vi "Initialize HMM Model.vi"(10 "M #observed states":i32=2, 11 "N #hidden states":i32=2) -> (3 "Init HMM":T1)   [LabVIEW 2014, in "HMM.lvlib"]
doc: "Generates the inital HMM a, b and Pi. The probability is random."
uses:
  HMM.lvlib
  Control/HMM Cluster.ctl
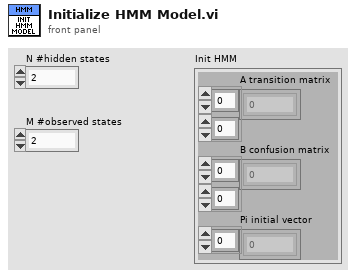
[diagram p1: front panel]
types:
  T1 = typedef "HMM.lvlib/HMM Cluster.ctl" = cluster{"A transition matrix":dbl[][], "B confusion matrix":dbl[][], "Pi initial vector":dbl[]}
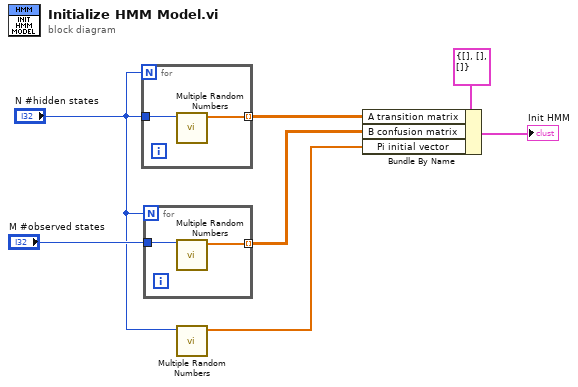
[diagram p0: block diagram]
diagram:
  n1 = for {
    N: "N #hidden states" -> [_]
    tunnel: "N #hidden states" -> [w9]
    tunnel: [w8] -> w5 mode=indexing
    n2 = call "Multiple Random Numbers.vi"("No. of rands"=w9) -> ("Random numbers"=w8:dbl[])  [unwired: 10 in]
  }
  n3 = for {
    N: "N #hidden states" -> [_]
    tunnel: "M #observed states" -> [w11]
    tunnel: [w10] -> w3 mode=indexing
    n4 = call "Multiple Random Numbers.vi"("No. of rands"=w11) -> ("Random numbers"=w10:dbl[])  [unwired: 10 in]
  }
  n5 = call "Multiple Random Numbers.vi"("No. of rands"="N #hidden states") -> ("Random numbers"=w1:dbl[])  [unwired: 10 in]
  n6 = Bundle By Name(cluster=T1 {"A transition matrix"=[], "B confusion matrix"=[], "Pi initial vector"=[]} ("Init lambda"), "A transition matrix"=w5, "B confusion matrix"=w3, "Pi initial vector"=w1) -> (→"Init HMM":T1)
